vi "Main_VI_1.vi"() -> ()   [LabVIEW 2020]
panel:
  in  "정지":bool
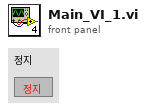
[diagram p1: front panel]
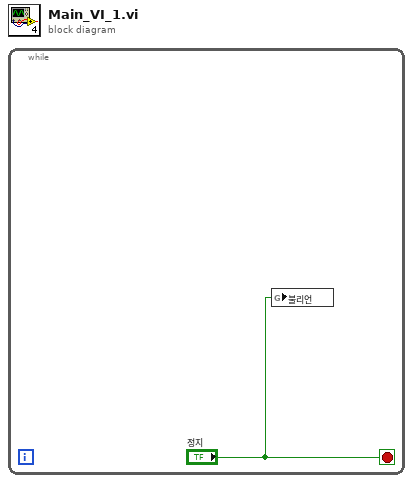
[diagram p0: block diagram]
diagram:
  n1 = while {
    stop <- "정지" stop-if-true
    n2 = global write "TEST_글로벌.vi" "불리언"("정지") -> ()
  }
